vi "Conversion between FXP and Integer.vi"() -> ()   [LabVIEW 2023]
doc: "Demonstrates how to use the DFD FXP Convert Integer to FXP VI and the DFD FXP Convert FXP to Integer VI to convert a fixed-point number to an integer number and vice versa.\n\nComplete the following steps to use this VI.\n1) Specify a floating-point number in the <B>Floating-Point Number</B> input.\n2) Specify the <B>Quantizer</B> settings.\n3) Run the VI.\n4) Observe the resulting Fixed-Point Number and Integer Value.\n5) Examine the block diagram to learn how to use the DFD FXP Convert Integer to FXP VI and the DFD FXP Convert FXP to Integer VI."
uses:
  <vilib>/addons/Digital Filter Design/_Objects.llb/DFD Quantization Settings.ctl
  <vilib>/addons/Digital Filter Design/_Objects.llb/DFD Quantization Sources.ctl
  <vilib>/addons/Digital Filter Design/FXPLib.llb/DFD FXP to I16 (scalar).vi
  <vilib>/addons/Digital Filter Design/FXPLib.llb/DFD I16 to FXP (scalar).vi
  <vilib>/addons/Digital Filter Design/NI_DigFilterLicensed.lvlib
panel:
  in  "Quantizer":T1={"source"=0, "wl"=16, "iwl"=1, "overflow mode"=enum."Wrap", "rounding mode"=enum."Truncation", "signed?"=TRUE} {"source" items=["Coefficients a/k"=0, "Coefficients b/v"=7, "Input"=1, "Output"=2, "Multiplicand"=3, "Product"=4, "Sum"=5, "Delay"=6]}
  out "Integer Value":i16
  out "Fixed-Point Number":dbl
  in  "Floating-Point Number":dbl=0.2321
  # "Select Help>>Show Context Help and move the cursor over the VI icon for more information."
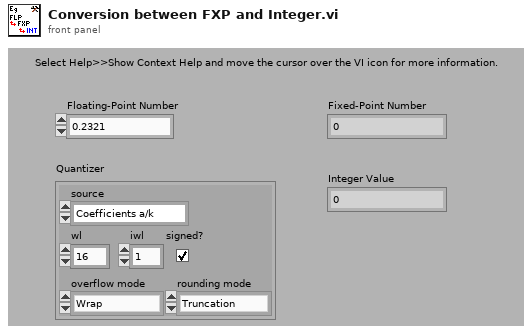
[diagram p1: front panel]
types:
  T1 = typedef "NI_DigFilterLicensed.lvlib/DFD Quantization Settings.ctl" = cluster{"source":T2, "wl":i16, "iwl":i16, "overflow mode":enum16{"Saturation", "Wrap"}, "rounding mode":enum16{"Nearest", "Truncation"}, "signed?":bool}
  T2 = typedef "NI_DigFilterLicensed.lvlib/DFD Quantization Sources.ctl" = u16
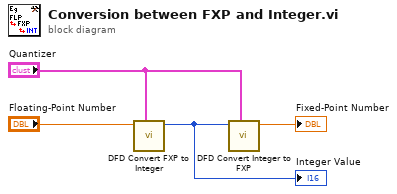
[diagram p0: block diagram]
diagram:
  n1 = call-poly <vilib>:"DFD Convert FXP to Integer.vi"("quantization settings"="Quantizer", "FXP value"="Floating-Point Number") -> ("I16"=w3:i16)  [unwired: 1 in, 8 out]
  "Integer Value" <- w3
  n2 = call-poly <vilib>:"DFD Convert Integer to FXP.vi"("quantization settings"="Quantizer", "I16"=w3) -> ("FXP value"=→"Fixed-Point Number":dbl)  [unwired: 1 in, 8 out]
